vi "17-tcoupl_sens.vi"(2 "this":i32, 3 "button":i32, 4 "Cluster":T1={"Auto1"=TRUE, "Auto2"=TRUE, "Rel1"=FALSE, "Rel2"=FALSE, "Filt1"=FALSE, "Filt2"=FALSE, "Rate"=enum."Slow", "Range1"=enum."10mV", "Range2"=enum."100mV", "Filt3"=FALSE, "Filt4"=FALSE, "Rel temp 1"=FALSE, "Analog1"=FALSE, "Analog2"=FALSE, "Analog temp 1"=FALSE, "Digital1"=FALSE, "Digital2"=FALSE, "Digital temp 1 "=FALSE, "Window1"=enum."None", "Window2"=enum."None", "Window temp 1"=enum."None", "RDGS1"="010", "RDGS2"="010", "RDGS temp 1"="010", "Type_type1"=TRUE, "Type_type2"=TRUE, "Type_type temp 1"=TRUE, "LSync"=FALSE, "Unit"=enum."C", "Sens"=TRUE, "Type tcoupl"=enum."J", "Junc"=TRUE, "prevState"=0, "Rel temp 2"=FALSE, "Analog temp 2"=FALSE, "Digital temp 2"=FALSE, "Type_type temp 2"=TRUE, "RDGS temp 2"="010", "Window temp 2"=enum."None", "address"="0"}) -> (0 "next state":i32, 1 "Cluster 2":T1)   [LabVIEW 2017]
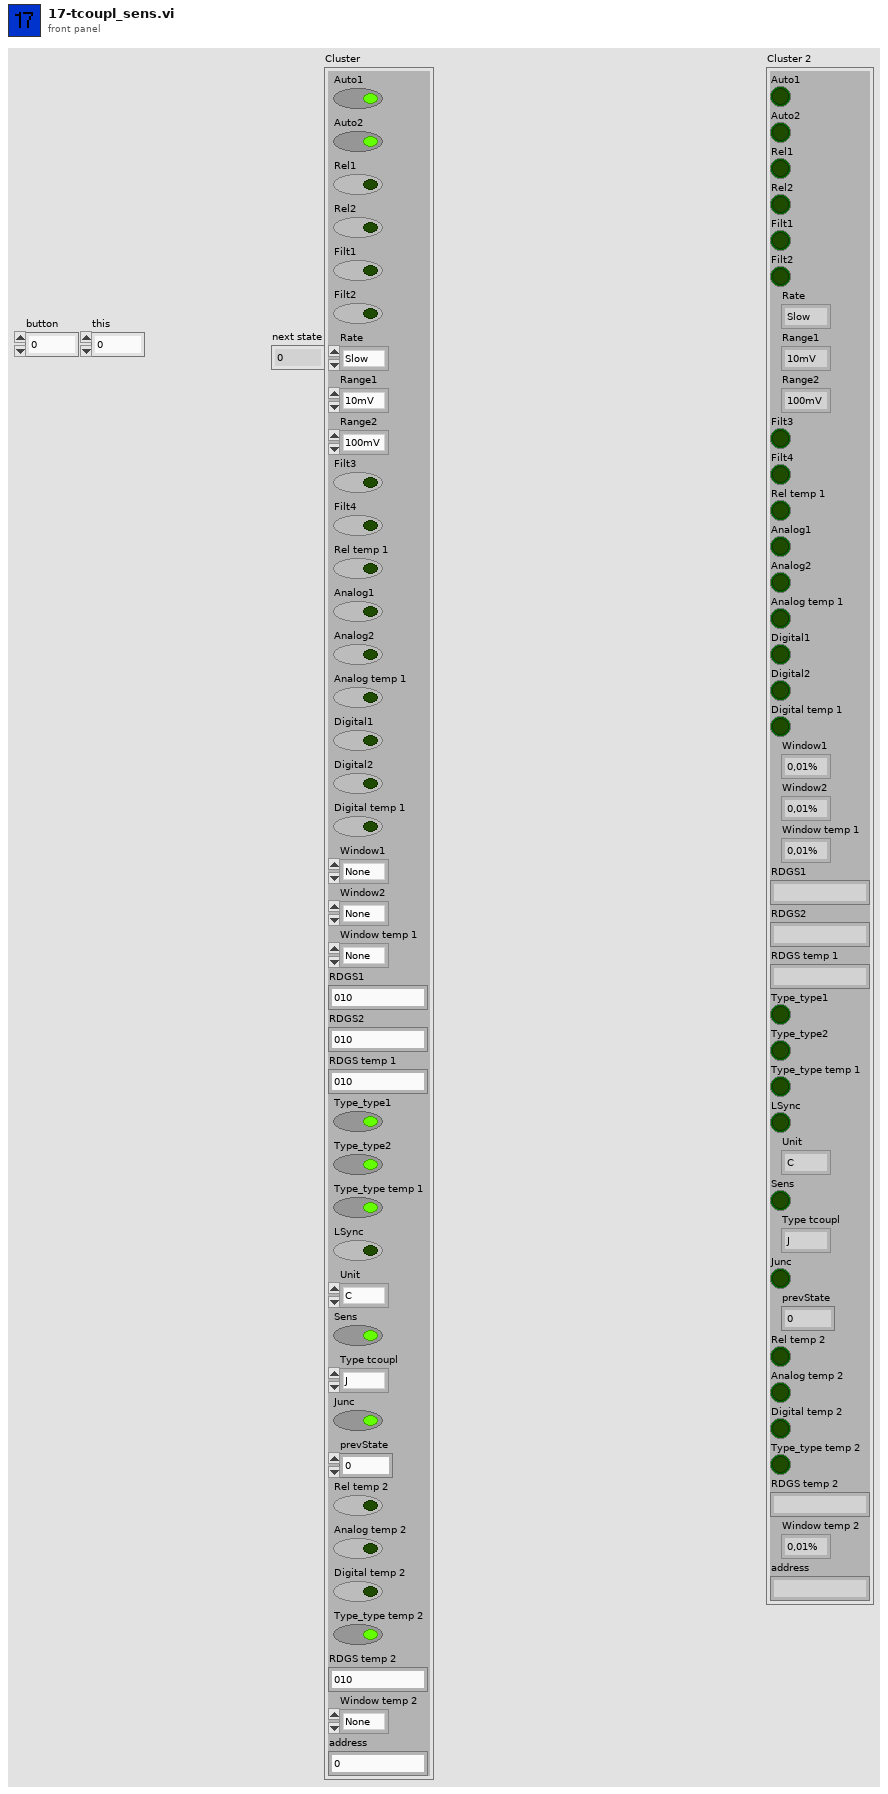
[diagram p1: front panel]
types:
  T1 = cluster{"Auto1":bool, "Auto2":bool, "Rel1":bool, "Rel2":bool, "Filt1":bool, "Filt2":bool, "Rate":enum16{"Slow", "Fast", "Med"}, "Range1":enum16{"10mV", "100mV", "1V", "10V", "100V"}, "Range2":enum16{"100mV", "1V", "10V"}, "Filt3":bool, "Filt4":bool, "Rel temp 1":bool, "Analog1":bool, "Analog2":bool, "Analog temp 1":bool, "Digital1":bool, "Digital2":bool, "Digital temp 1 ":bool, "Window1":enum16{"0,01%", "0,1%", "1%", "10%", "None"}, "Window2":enum16{"0,01%", "0,1%", "1%", "10%", "None"}, "Window temp 1":enum16{"0,01%", "0,1%", "1%", "10%", "None"}, "RDGS1":string, "RDGS2":string, "RDGS temp 1":string, "Type_type1":bool, "Type_type2":bool, "Type_type temp 1":bool, "LSync":bool, "Unit":enum16{"C", "K", "F"}, "Sens":bool, "Type tcoupl":enum16{"J", "K", "T", "E", "R", "S", "B", "N"}, "Junc":bool, "prevState":i32, "Rel temp 2":bool, "Analog temp 2":bool, "Digital temp 2":bool, "Type_type temp 2":bool, "RDGS temp 2":string, "Window temp 2":enum16{"0,01%", "0,1%", "1%", "10%", "None"}, "address":string}
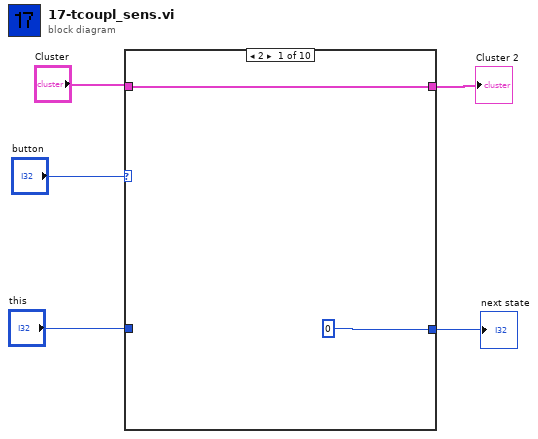
[diagram p0: block diagram]
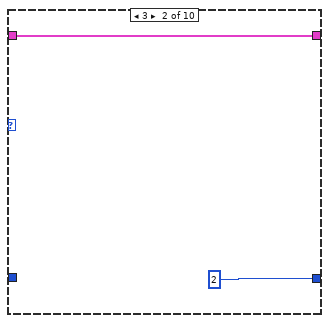
[diagram p2: hidden frame]
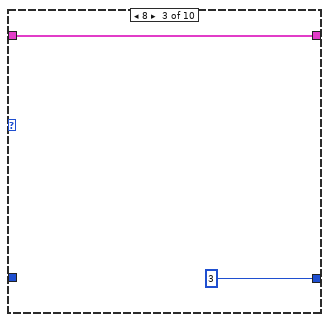
[diagram p3: hidden frame]
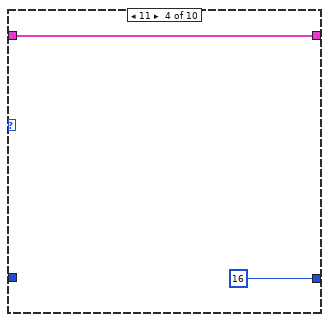
[diagram p4: hidden frame]
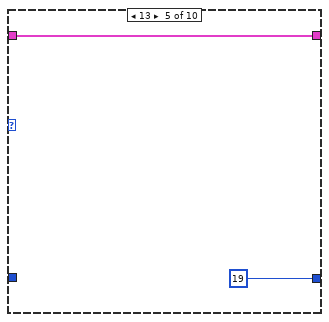
[diagram p5: hidden frame]
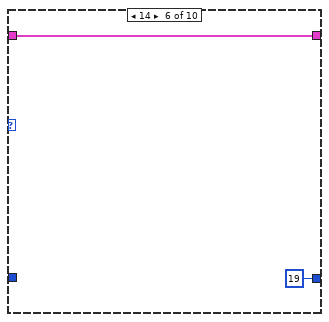
[diagram p6: hidden frame]
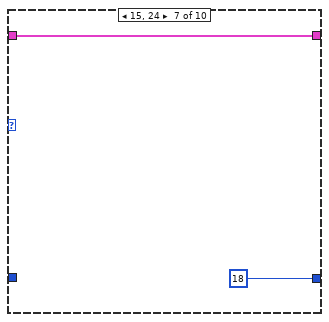
[diagram p7: hidden frame]
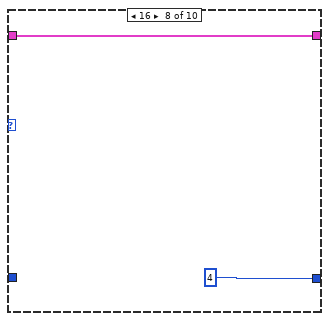
[diagram p8: hidden frame]
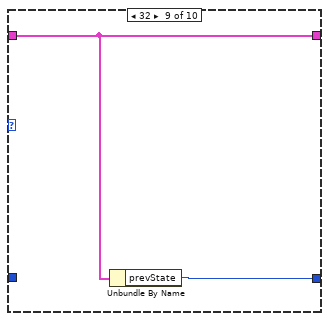
[diagram p9: hidden frame]
diagram:
  n1 = case shown="2" "button" {
    tunnel: [0 ("this") 2 3 16 ("this") 19 ("this") 19 ("this") 18 ("this") 4 w22 w24] -> w3
    tunnel: "this" -> [_ _ _ _ _ _ _ _ _ w24]
    tunnel: "Cluster" -> [w7 w8 w10 w13 w15 w17 w19 w20 w23 w25]
    tunnel: [w7 w8 w10 w13 w15 w17 w19 w20 w23 w25] -> w1
    frame 2 {
    }
    frame 3 {
    }
    frame 8 {
    }
    frame 11 {
    }
    frame 13 {
    }
    frame 14 {
    }
    frame 15, 24 {
    }
    frame 16 {
    }
    frame 32 {
      n2 = Unbundle By Name(w23) -> ("prevState"=w22:i32)
    }
    frame Default {
    }
  }
  "next state" <- w3
  "Cluster 2" <- w1
